vi "AL_포맷정보_변환_TEST.vi"() -> ()   [LabVIEW 2017]
panel:
  out "부호없는 바이트 배열":u8[](array[numeric])
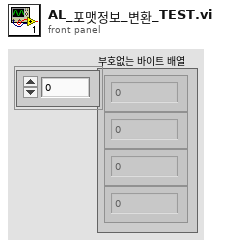
[diagram p1: front panel]
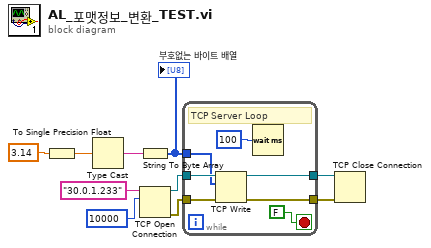
[diagram p0: block diagram]
diagram:
  n1 = To Single Precision Float(number=3.14) -> (single precision float=w2:sgl)
  n2 = Type Cast(x=w2) -> (*(type *) &x=w1:string)  [unwired: 1 in]
  n3 = String To Byte Array(string=w1) -> (unsigned byte array=w8:u8[])
  "부호없는 바이트 배열" <- w8
  n4 = TCP Open Connection(address="30.0.1.233" ("주소"), remote port or service name=u16 10000 ("원격 포트 또는 서비스 이름")) -> (connection ID=w5:refnum<k5>, error out=w4:errorcluster)  [unwired: 3 in]
  n5 = while {
    tunnel: w5 -> [w16]
    tunnel: w4 -> [w15]
    tunnel: [w14] -> w10
    tunnel: [w13] -> w9
    tunnel: w8 -> [w12]
    stop <- FALSE stop-if-true
    # "TCP Server Loop"
    n6 = TCP Write(connection ID=w16, data in=w12, error in (no error)=w15) -> (connection ID out=w13:refnum<k5>, error out=w14:errorcluster)  [unwired: 2 out]
    n7 = Wait (ms)(milliseconds to wait=u32 100) -> ()  [unwired: 1 out]
  }
  n8 = TCP Close Connection(connection ID=w9, error in (no error)=w10) -> ()  [unwired: 3 out]
